vi "Min Read Array.vi"(8 "error in":errorcluster, 11 "Min Temperature Limit in":refnum<class "Temperature Limit.lvclass">) -> (0 "error out":errorcluster, 1 "Changed or First Call?":bool, 2 "Temperature Min SP":dbl[](array[numeric]), 3 "Min Temperature Limit out":refnum<class "Temperature Limit.lvclass">)   [LabVIEW 2023, in "Temperature Limit.lvclass"]
uses:
  Temperature Limit.lvclass
  Parents/Limit/Limit.lvclass
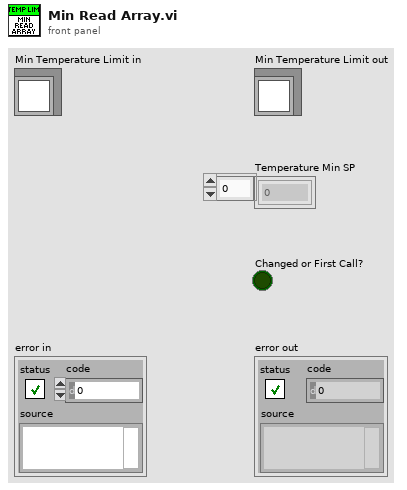
[diagram p1: front panel]
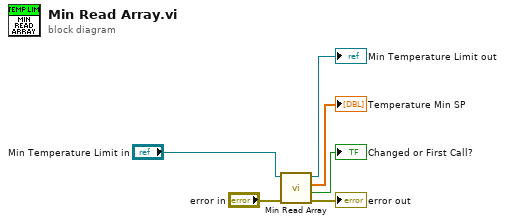
[diagram p0: block diagram]
diagram:
  n1 = call-parent "Min Read Array.vi"("error in"="error in", "Min Limit in"="Min Temperature Limit in") -> ("error out"=→"error out":errorcluster, "Changed or First Call?"=→"Changed or First Call?":bool, "Current Min SP"=→"Temperature Min SP":dbl[], "Min Limit out"=→"Min Temperature Limit out":refnum<class "Temperature Limit.lvclass">)  [unwired: 6 in]
